vi "Abort.vi"(11 "Actor":refnum<class "Actor.lvclass">) -> (3 "Actor":refnum<class "Actor.lvclass">)   [LabVIEW 2020, in "jettl.lvlib"]
uses:
  jettl.lvlib
  Message/Message.lvclass
  LifecycleEnum.ctl
  Actor/Actor.lvclass
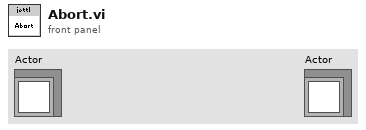
[diagram p1: front panel]
types:
  T1 = typedef "jettl.lvlib/LifecycleEnum.ctl" = enum16{"Initializing", "SettingUp", "Starting", "Running", "Stopping", "TearingDown", "Terminated", "Abort"}
  T2 = typedef "jettl.lvlib/BaseCluster.ctl" = cluster{"LifecycleEnum":T1, "MainCluster":T3, "SelfActorCluster":T4, "MediatorActorCluster":T4, "ComponentActorClusterMap":T9}
  T3 = typedef "jettl.lvlib/MainCluster.ctl" = cluster{"PreSetupClusterQueue":refnum<queue>, "BeginSetupQueue":refnum<queue>, "PostSetupClusterQueue":refnum<queue>, "BeginLoopQueue":refnum<queue>}
  T4 = typedef "jettl.lvlib/ActorCluster.ctl" = cluster{"MessagesCluster":T5, "Alias":string, "ActorTypeEnum":T8, "MessageClusterDVREvent":refnum<user-event>, "EventRegistrationRef":refnum<event-registration>, "VIRef":refnum<vi>}
  T5 = typedef "jettl.lvlib/MessagesCluster.ctl" = cluster{"ListenMessageSet":T6, "TellSelfMessageSet":T6, "TellMediatorMessageSet":T6, "TellComponentMessageSetMap":T7}
  T6 = typedef "jettl.lvlib/MessageSet.ctl" = set{refnum<class "Message.lvclass">}
  T7 = typedef "jettl.lvlib/TellComponentMessageSetMap.ctl" = map{string, T6}
  T8 = typedef "jettl.lvlib/ActorTypeEnum.ctl" = enum16{"Mediator", "Component"}
  T9 = typedef "jettl.lvlib/ComponentActorClusterMap.ctl" = map{string, T4}
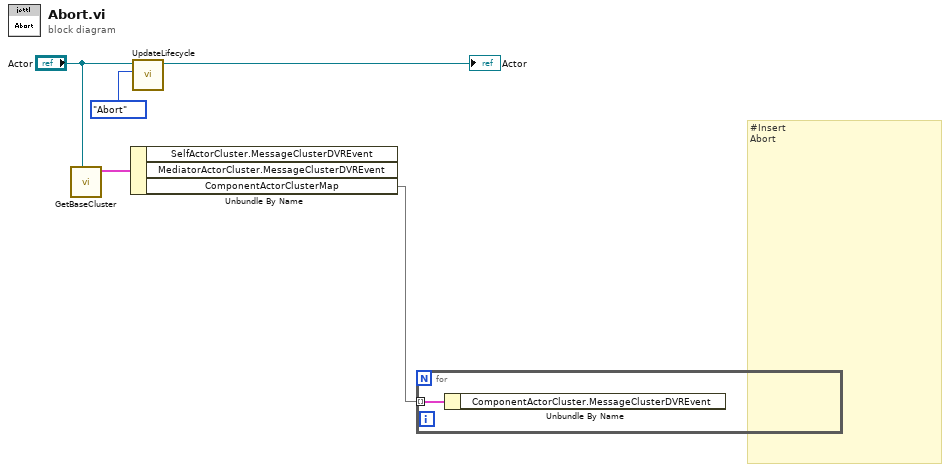
[diagram p0: block diagram]
diagram:
  # "#Insert\nAbort"
  n1 = call-dynamic "GetBaseCluster.vi"("Actor"="Actor") -> ("BaseCluster"=w4:T2)  [unwired: 10 in]
  n2 = Unbundle By Name(w4) -> ("SelfActorCluster.MessageClusterDVREvent"=w1:refnum<user-event>, "MediatorActorCluster.MessageClusterDVREvent"=w2:refnum<user-event>, "ComponentActorClusterMap"=w3:T9)
  n3 = call "UpdateLifecycle.vi"("Lifecycle"=LifecycleEnum."Abort", "Actor"="Actor") -> ("Actor"=→"Actor":refnum<class "Actor.lvclass">)  [unwired: 9 in]
  n4 = for {
    tunnel: w3 -> [w9] mode=indexing
    n5 = Unbundle By Name(w9) -> ("ComponentActorCluster.MessageClusterDVREvent"=w8:refnum<user-event>)
  }
